vi "rand124.vi"() -> (0 "rand":u32)   [LabVIEW 2023]
uses:
  <vilib>/numeric/Random Number (Range) I64.vi
  <vilib>/numeric/sub_Random U32.vi
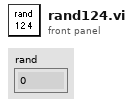
[diagram p1: front panel]
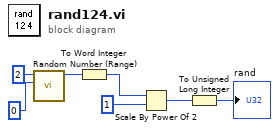
[diagram p0: block diagram]
diagram:
  n1 = call-poly <vilib>:"Random Number (Range).vi"("lower bound (-100)"=i64 0, "upper bound (100)"=i64 2) -> ("number"=w6:i64)  [unwired: 9 in]
  n2 = To Word Integer(number=w6) -> (16bit integer=w7:i16)
  n3 = Scale By Power Of 2(n=w7, x=i64 1 ("lower bound (-100)")) -> (x*2^n=w2:i64)
  n4 = To Unsigned Long Integer(number=w2) -> (unsigned 32bit integer=→"rand":u32)
